vi "Pressure_Release.vi"() -> ()   [LabVIEW 2014]
uses:
  <vilib>/rvi/Emulation/niFpgaGetClockAttributes.vi
  <vilib>/rvi/Emulation/niFpgaSctlEmulationGetInTimedLoop.vi
  <vilib>/rvi/Emulation/niFpgaEmulationReportErrorSimple.vi
  <vilib>/rvi/eio/common/nirviEmuTemplateMethod_errors.vi
  <vilib>/rvi/Emulation/niFpgaCriticalErrorInLSC.vi
  <vilib>/eio/EIONode/EIONode.xnode
panel:
  out "Pressure_Tank":fxp<+/-,26,5>
  in  "TankHi":fxp<+/-,20,5>
  in  "TankLo":fxp<+/-,20,5>
  in  "Leak test on?":bool
  out "Active?":bool
  in  "PR Test":bool
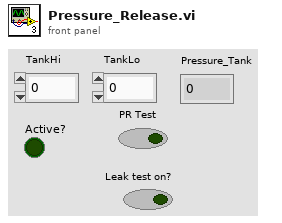
[diagram p1: front panel]
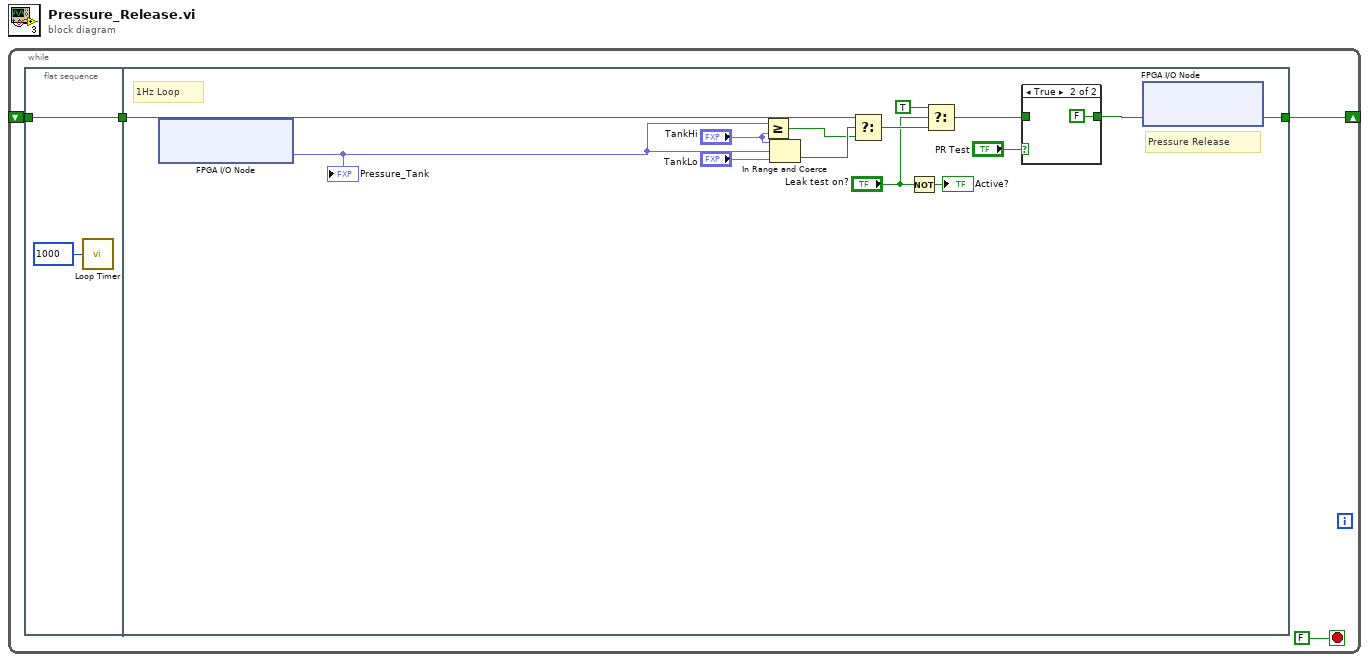
[diagram p0: block diagram]
diagram:
  n1 = while {
    shift-right: [w2] -> _
    shift-left: _ -> [w3]
    stop <- FALSE ("stop") stop-if-true
    n2 = flat-sequence {
      tunnel: [w5] -> w1
      tunnel: w3 -> [w5]
      tunnel: w1 -> [w19]
      tunnel: [w9] -> w2
      frame #0 {
        n3 = call "Loop Timer"("Count(mSec)"=u32 1000) -> ()  [unwired: 1 out]
      }
      frame #1 {
        # "Pressure Release"
        # "1Hz Loop"
        n4 = xnode "FPGA I/O Node"() -> ("Pressure_Tank"=w11:fxp<+/-,26,5>)  [unwired: 2 in, 2 out]
        "Pressure_Tank" <- w11
        n5 = Greater Or Equal?(x=w11, y="TankHi") -> (x >= y?=w7:bool)
        n6 = In Range and Coerce(upper limit="TankHi", x=w11, lower limit="TankLo") -> (In Range?=w18:bool)  [unwired: 1 out]
        n7 = Select(t=w19, s=w18, f=w7) -> (s? t:f=w15:bool)
        n8 = Not(x="Leak test on?") -> (.not. x?=→"Active?":bool)
        n9 = Select(t=TRUE, s="Leak test on?", f=w15) -> (s? t:f=w10:bool)
        n10 = case shown="True" "PR Test" {
          tunnel: w10 -> [w20 _]
          tunnel: [w20 FALSE ("f")] -> w9
          frame False {
          }
          frame True {
          }
        }
        n11 = xnode "FPGA I/O Node"("Tank-PR_SV"=w9) -> ()  [unwired: 2 in, 2 out]
      }
    }
  }
